vi "Test Process Log Running Lifecycle State.vi"(8 "error in (no error)":errorcluster, 11 "Process Test In":refnum<class "Process Dev Test.lvclass">) -> (0 "error out":errorcluster, 3 "Process Test Out":refnum<class "Process Dev Test.lvclass">)   [LabVIEW 2020, in "Process Dev Test.lvclass"]
uses:
  Process Dev Test.lvclass
  C:/Program Files (x86)/National Instruments/LabVIEW 2020/vi.lib/Astemes/LUnit/Test Case.lvclass
  source/Framework Test Suite/Mock Log Handler/Mock Log Handler.lvclass
  C:/Git/astemes-triarc-framework/source/Framework/Logging/Logging.lvclass
  source/Framework/Process/Process.lvclass/Process.ctl
  <vilib>/Astemes/LUnit/Test Case.lvclass/Test Case.ctl
  <vilib>/Astemes/LUnit/LUnit Assertion Result.lvclass/LUnit Assertion Result.ctl
  <vilib>/Astemes/LUnit/LUnit Test Case Result.lvclass/LUnit Test Case Result.ctl
  <vilib>/Astemes/LUnit/LUnit Method Result.lvclass/LUnit Method Result.ctl
  63cd48a4-71ab-406d-8512-4a07cc0c0a64.vi
  source/Framework/Process/Public/Lifecycle/Get Lifecycle State.vi
  source/Framework/Process/Protected/Messaging/Send Message.vi
  source/Framework/Process/Private/SubVIs/Wait for finish.vi
  source/Framework/Process/Private/SubVIs/Set Lifecycle State.vi
  <vilib>/Astemes/LUnit/Palette/Pass.vi
  <vilib>/Astemes/LUnit/Palette/Fail.vi
  <vilib>/Astemes/LUnit/Compare Variants.vi
  <vilib>/Astemes/LUnit/Describe Comparison.vi
  <vilib>/Astemes/LUnit/Set Assertion Type.vi
  <vilib>/Utility/error.llb/Clear Errors.vi
  source/Framework/Process/Private/SubVIs/Handle Debug Data.vi
  <vilib>/Astemes/LUnit/Add test result.vi
  <vilib>/Astemes/LUnit/LUnit Write Passed.vi
  <vilib>/Astemes/LUnit/LUnit Write Message.vi
  <vilib>/Astemes/LUnit/LUnit Write Description.vi
  <vilib>/Astemes/LUnit/Variant to string.vi
  <vilib>/Astemes/LUnit/LUnit Write Assertion Type.vi
  source/Framework/Logging/Log Debug.vi
  <vilib>/AdvancedString/1D String Array to Delimited String.vi
  <vilib>/Utility/High Resolution Relative Seconds.vi
  <vilib>/Astemes/LUnit/LUnit Record Assertion Result.vi
  <vilib>/Astemes/LUnit/LUnit Aggregate Assertion Results.vi
  <vilib>/Astemes/LUnit/Assertion Result/LUnit Read Status.vi
  <vilib>/Astemes/LUnit/LUnit Read Message.vi
  <vilib>/Astemes/LUnit/LUnit Read Description.vi
  <vilib>/Astemes/LUnit/Method Result/LUnit Merge Status.vi
  <vilib>/Astemes/LUnit/LUnit Concatenate result strings.vi
  <vilib>/Utility/error.llb/Error Cluster From Error Code.vi
  source/Framework/Process/Public/Read Name.vi
  <vilib>/Utility/Data Type/Get Type Information.vi
  <vilib>/Utility/LVClass/Get LV Class Name.vi
  <vilib>/Astemes/LUnit/LUnit Assertion Result.lvclass
  source/Framework/Process/Process.lvclass
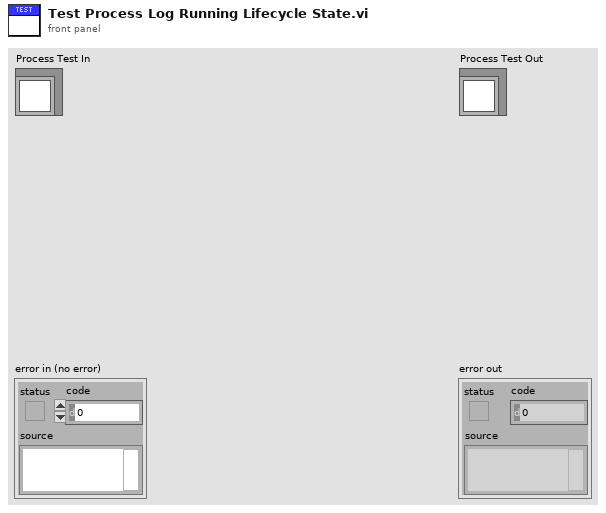
[diagram p1: front panel]
types:
  T1 = typedef "Mock Log Handler.lvclass/Log Entry.ctl" = cluster{"Level":string, "Source":string, "Message":string}
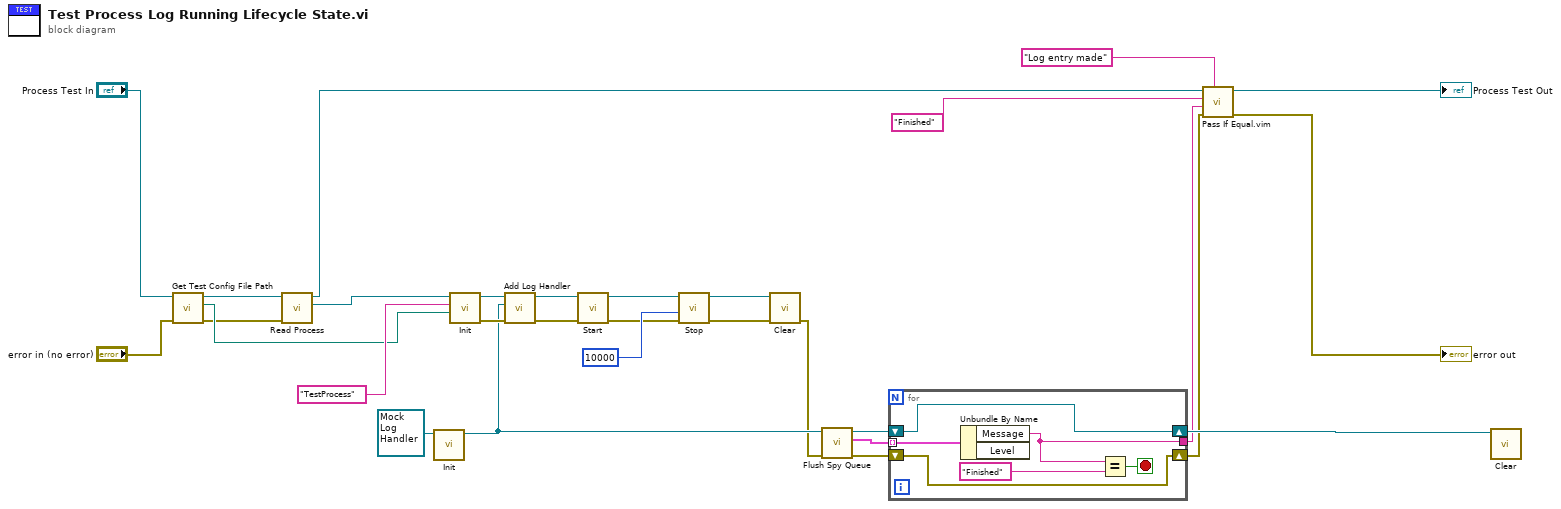
[diagram p0: block diagram]
diagram:
  n1 = call "Get Test Config File Path.vi"("error in (no error)"="error in (no error)", "Process Test In"="Process Test In") -> ("error out"=w18:errorcluster, "Test config path"=w21:path, "Process Test Out"=w20:refnum<class "Process Dev Test.lvclass">)  [unwired: 7 in]
  n2 = call "Read Process.vi"("error in (no error)"=w18, "Process Test in"=w20) -> ("Process.lvclass"=w19:refnum<class "Process.lvclass">, "Process Test out"=w16:refnum<class "Process Dev Test.lvclass">)  [unwired: 7 in, 1 out]
  n3 = call-dynamic "Init.vi"("Mock Log Handler In"=refnum<class "Mock Log Handler.lvclass"> refnum) -> ("Mock Log Handler Out"=w9:refnum<class "Mock Log Handler.lvclass">)  [unwired: 9 in, 1 out]
  n4 = call-dynamic "Init.vi"("Config File Path"=w21, "Name"="TestProcess", "Process In"=w19) -> ("error out"=w30:errorcluster, "Process Out"=w14:refnum<class "Process.lvclass">)  [unwired: 7 in]
  n5 = call "Add Log Handler.vi"("error in (no error)"=w30, "Log Handler"=w9, "Process In"=w14) -> ("error out"=w24:errorcluster, "Process Out"=w29:refnum<class "Process.lvclass">)  [unwired: 7 in]
  n6 = call "Start.vi"("error in (no error)"=w24, "Process In"=w29) -> ("error out"=w6:errorcluster, "Process Out"=w28:refnum<class "Process.lvclass">)  [unwired: 7 in, 1 out]
  n7 = call "Stop.vi"("error in (no error)"=w6, "timeout in ms (-1)"=10000, "Process In"=w28) -> ("error out"=w4:errorcluster, "Process Out"=w27:refnum<class "Process.lvclass">)  [unwired: 6 in, 1 out]
  n8 = call-dynamic "Clear.vi"("error in (no error)"=w4, "Process In"=w27) -> ("error out"=w3:errorcluster)  [unwired: 9 in]
  n9 = call "Flush Spy Queue.vi"("error in (no error)"=w3, "Mock Log Handler in"=w9) -> ("error out"=w2:errorcluster, "remaining elements"=w1:T1[], "Mock Log Handler out"=w8:refnum<class "Mock Log Handler.lvclass">)  [unwired: 7 in]
  n10 = for {
    shift-right: [w36] -> w12
    shift-left: w8 -> [w36]
    shift-right: [w35] -> w7
    shift-left: w2 -> [w35]
    tunnel: [w33] -> w11
    tunnel: w1 -> [w32] mode=indexing
    stop <- w31 stop-if-true
    n11 = Unbundle By Name(w32) -> ("Message"=w33:string)  [unwired: 1 out]
    n12 = Equal?(x=w33, y="Finished") -> (x = y?=w31:bool)
  }
  n13 = call "Pass If Equal.vim"("Description"="Log entry made", "error in (no error)"=w7, "Actual"=w11, "Expected"="Finished", "LUnit Test Case In"=w16) -> ("error out"=→"error out":errorcluster, "LUnit Test Case Out"=→"Process Test Out":refnum<class "Process Dev Test.lvclass">)  [unwired: 5 in]
  n14 = call-dynamic "Clear.vi"("Mock Log Handler In"=w12) -> ()  [unwired: 10 in, 1 out]
